vi "Add LINBus Received Frames.vi"(8 "error in (no error)":errorcluster, 10 "LIN Frames":T1[](array[typedef]) {"event ID" format="%x"; "payload" format="%x"; "timestamp" format="%<%.7X\n%x>T"; "type" items=["LIN Data"=64, "LIN Bus Error"=65, "LIN No Response"=66, "Delay"=224, "Log Trigger"=225, "Start Trigger"=226]; "identifier" format="%x"}, 11 "Load Calculator in":refnum<class "GenBus_Load_Calculator.lvclass">) -> (0 "error out":errorcluster, 3 "Load Calculator out":refnum<class "GenBus_Load_Calculator.lvclass">)   [LabVIEW 2019, in "XNET-Bus-Load-Calculator.lvlib"]
uses:
  XNET-Bus-Load-Calculator.lvlib
  GenBus/GenBus_Load_Calculator.lvclass
  <vilib>/xnet/xnet.llb/XNET Frame LIN.ctl
  <vilib>/xnet/xnet.llb/XNET Frame Type LIN.ctl
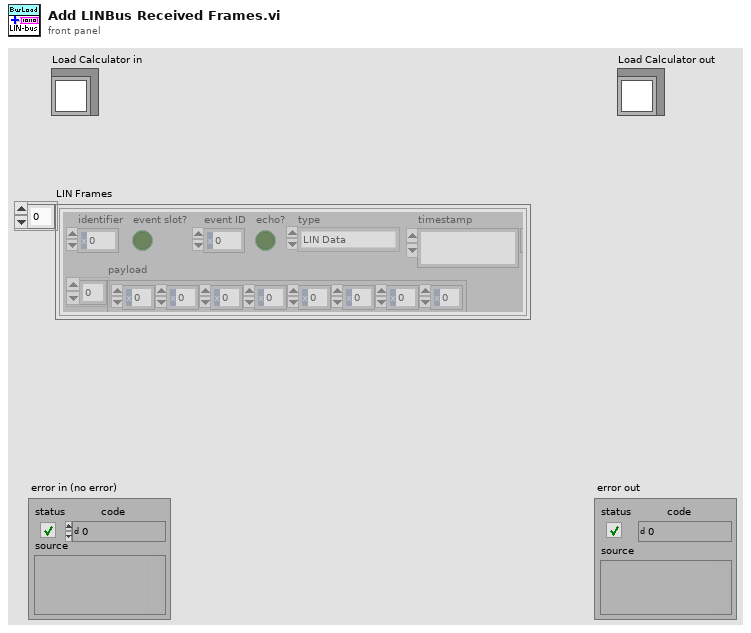
[diagram p1: front panel]
types:
  T1 = typedef "XNET Frame LIN.ctl" = cluster{"timestamp":timestamp, "payload":u8[], "identifier":u32, "type":T2, "event ID":u8, "event slot?":bool, "echo?":bool}
  T2 = typedef "XNET Frame Type LIN.ctl" = u8
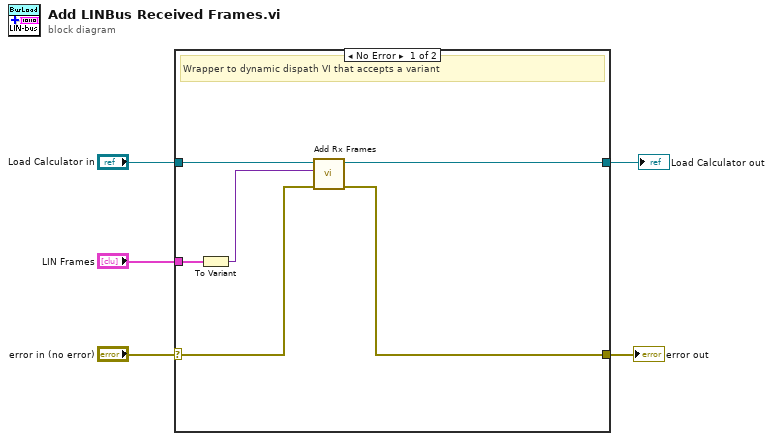
[diagram p0: block diagram]
diagram:
  n1 = case shown="No Error" "error in (no error)" {
    selector: "error in (no error)" -> [w9 w13]
    tunnel: [w6 w13] -> w1
    tunnel: "LIN Frames" -> [w8 _]
    tunnel: "Load Calculator in" -> [w11 w12]
    tunnel: [w10 w12] -> w2
    frame No Error {
      # "Wrapper to dynamic dispath VI that accepts a variant"
      n2 = To Variant(anything=w8) -> (Variant=w7:variant)
      n3 = call-dynamic "Add Rx Frames.vi"("error in (no error)"=w9, "Frames"=w7, "GenBus_Load_Calculator in"=w11) -> ("error out"=w6:errorcluster, "GenBus_Load_Calculator out"=w10:refnum<class "GenBus_Load_Calculator.lvclass">)  [unwired: 7 in]
    }
    frame Error {
    }
  }
  "error out" <- w1
  "Load Calculator out" <- w2
